vi "Is Data Ready.vi"(8 "error in (no error)":errorcluster, 11 "DAQmx Digitizer in":refnum<class "DAQmx Synthesizer.lvclass">) -> (0 "error out":errorcluster, 1 "Data ready":bool, 2 "Availiable Samples":u32, 3 "DAQmx Digitizer out":refnum<class "DAQmx Synthesizer.lvclass">)   [LabVIEW 2021]
uses:
  DAQmx Synthesizer.lvclass
  DAQmx Synthesizer.lvclass/DAQmx Synthesizer.ctl
  <resource>/objmgr/daqmx.rc
  C:/GitHub/NHMFL_Core/Libraries/NI-DAQ/DAQmx Digitizer/DAQmx Digitizer.lvclass
  C:/GitHub/NHMFL_Core/Libraries/Instruments/Pulse Driver/Lockin Digitizer Driver/Lockin Digitizer Driver.lvclass
  C:/GitHub/NHMFL_Core/Libraries/Instruments/Pulse Driver/Pulse Driver.lvclass
  C:/GitHub/NHMFL_Core/Libraries/Instruments/Instrument Driver/Instrument Driver.lvclass
  C:/GitHub/NHMFL_Core/Libraries/NI-DAQ/DAQmx Synthesizer/DAQmx Synthesizer.lvclass
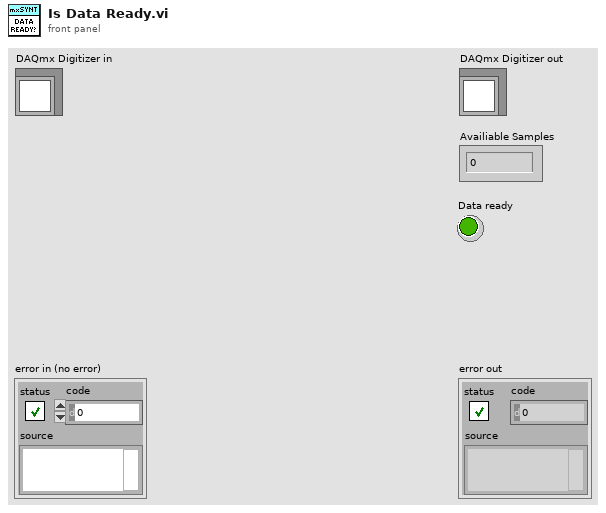
[diagram p1: front panel]
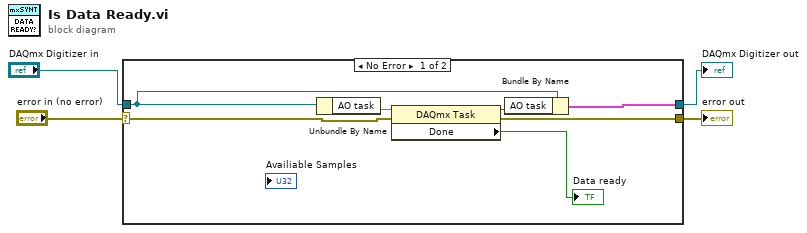
[diagram p0: block diagram]
diagram:
  n1 = case shown="No Error" "error in (no error)" {
    selector: "error in (no error)" -> [w6 w13]
    tunnel: [w11 w13] -> w2
    tunnel: [w10 w12] -> w1
    tunnel: "DAQmx Digitizer in" -> [w7 w12]
    frame No Error {
      n2 = Unbundle By Name(w7) -> ("AO task"=w8)
      n3 = property class="DAQmx Task"(reference=w8, error in=w6) -> (reference out=w9:refnum<k21>, error out=w11:errorcluster, "Done"=→"Data ready":bool)
      n4 = Bundle By Name(cluster=w7, "AO task"=w9) -> (w10:cluster{})
    }
    frame Error {
    }
  }
  "error out" <- w2
  "DAQmx Digitizer out" <- w1
